vi "GetParentDirectory.vi"(8 "error in":errorcluster caption="entrée d'erreur", 11 "VIPath":path) -> (0 "error out":errorcluster caption="sortie d'erreur", 3 "VIRelativePath":path, 5 "IsItDirectory?":bool)   [LabVIEW 2022 SP3, in "EClib functions.lvlib"]
doc: "Cette fonction renvoie le chemin du dossier contenant le VI spécifié en entrée"
uses:
  EClib functions.lvlib
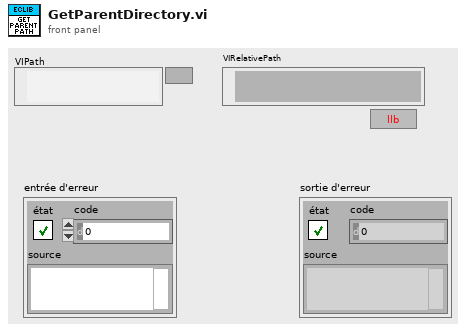
[diagram p1: front panel]
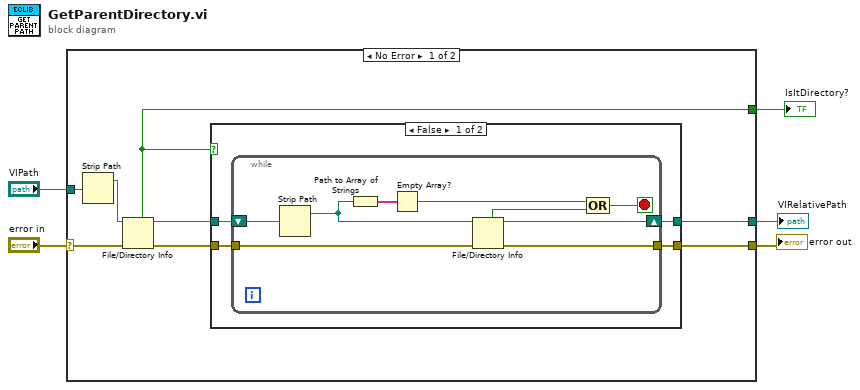
[diagram p0: block diagram]
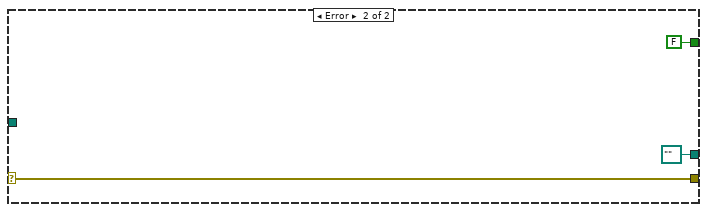
[diagram p3: hidden frame]
diagram:
  n1 = case shown="No Error" "error in" {
    selector: "error in" -> [w7 w29]
    tunnel: "VIPath" -> [w12 _]
    tunnel: [w10 path "" ("path out")] -> w4
    tunnel: [w9 FALSE ("directory")] -> w3
    tunnel: [w6 w29] -> w1
    frame No Error {
      n2 = Strip Path(path=w12) -> (stripped path=w13:path)  [unwired: 1 out]
      n3 = File/Directory Info(path=w13, error in=w7) -> (path out=w11:path, directory=w9:bool, error out=w8:errorcluster)  [unwired: 4 out]
      n4 = case shown="False" w9 {
        tunnel: w11 -> [w17 w28]
        tunnel: [w16 w28] -> w10
        tunnel: [w15 w27] -> w6
        tunnel: w8 -> [w14 w27]
        frame False {
          n5 = while {
            shift-right: [w25] -> w16
            shift-left: w17 -> [w26]
            tunnel: [w23] -> w15
            tunnel: w14 -> [w20]
            stop <- w24 stop-if-true
            n6 = Strip Path(path=w26) -> (stripped path=w22:path)  [unwired: 1 out]
            n7 = Path to Array of Strings(0:w22) -> (2:w21:string[])  [unwired: 1 out]
            n8 = Empty Array?(array=w21) -> (empty?=w19:bool)
            n9 = File/Directory Info(path=w22, error in=w20) -> (path out=w25:path, directory=w18:bool, error out=w23:errorcluster)  [unwired: 4 out]
            n10 = Compound Arithmetic op=OR(w19, w18) -> (w24:bool)
          }
        }
        frame True {
        }
      }
    }
    frame Error {
    }
  }
  "VIRelativePath" <- w4
  "IsItDirectory?" <- w3
  "error out" <- w1
